vi "AutoCrossSubVi.vi"(0 "AutoDriveSpeed":dbl, 1 "DistanceAutoLineToBar":dbl, 2 "BarToShootLine":dbl, 3 "DriveDistanceDeadband":dbl, 5 "DriveDistanceVDeadband":dbl, 7 "VDeadband":dbl, 9 "EncoderDevRef 2":T1, 12 "Deadband":dbl, 13 "String":string, 14 "EncoderDevRef":T1) -> ()   [LabVIEW 2015]
uses:
  AutoTask/Implementation/AutoTask Operations.ctl
  AutoTask/Implementation/AutoTask Setpoints.ctl
  <vilib>/Rock Robotics/SystemInterfaces/Encoder/FPGA_EncoderIdx.ctl
  <vilib>/Rock Robotics/WPI/Encoder/WPI_EncoderType.ctl
  <vilib>/Rock Robotics/SystemInterfaces/Counter/FPGA_CounterCtrSystemIndex.ctl
  <vilib>/Rock Robotics/WPI/Encoder/WPI_EncoderDevRef.ctl
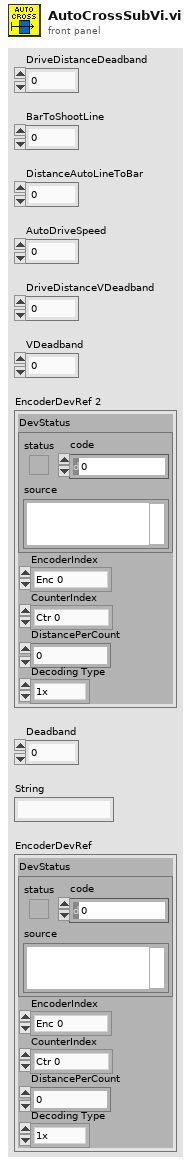
[diagram p1: front panel]
types:
  T1 = typedef "WPI_EncoderDevRef.ctl" = cluster{"DevStatus":errorcluster, "EncoderIndex":T2, "CounterIndex":T3, "DistancePerCount":dbl, "Decoding Type":T4}
  T2 = typedef "FPGA_EncoderIdx.ctl" = enum8{"Enc 0", "Enc 1", "Enc 2", "Enc 3", "Enc 4", "Enc 5", "Enc 6", "Enc 7", "Invalid"}
  T3 = typedef "FPGA_CounterCtrSystemIndex.ctl" = enum8{"Ctr 0", "Ctr 1", "Ctr 2", "Ctr 3", "Ctr 4", "Ctr 5", "Ctr 6", "Ctr 7", "Invalid"}
  T4 = typedef "WPI_EncoderType.ctl" = enum16{"1x", "2x", "4x"}
  T5 = typedef "AutoTask Setpoints.ctl" = cluster{"Operation":T6, "Setpoint":dbl, "Duration":dbl, "Speed":dbl, "Angle":dbl, "VDeadband":dbl, "Deadband":dbl, "DriveSpeed":dbl}
  T6 = typedef "AutoTask Operations.ctl" = enum16{"Reserve", "Read Current", "Immediate", "DriveDistance", "AutoShoot", "FaceForward", "AutoAlign", "AutoTurn", "DriveToLine", "DriveToIncline", "DriveTillFlat"}
  T7 = typedef "AutoTask Setpoints.ctl" = cluster{"Operation":T6, "Setpoint":dbl, "Duration":dbl, "Speed":dbl, "Angle":dbl, "VDeadband":dbl, "Deadband":dbl}
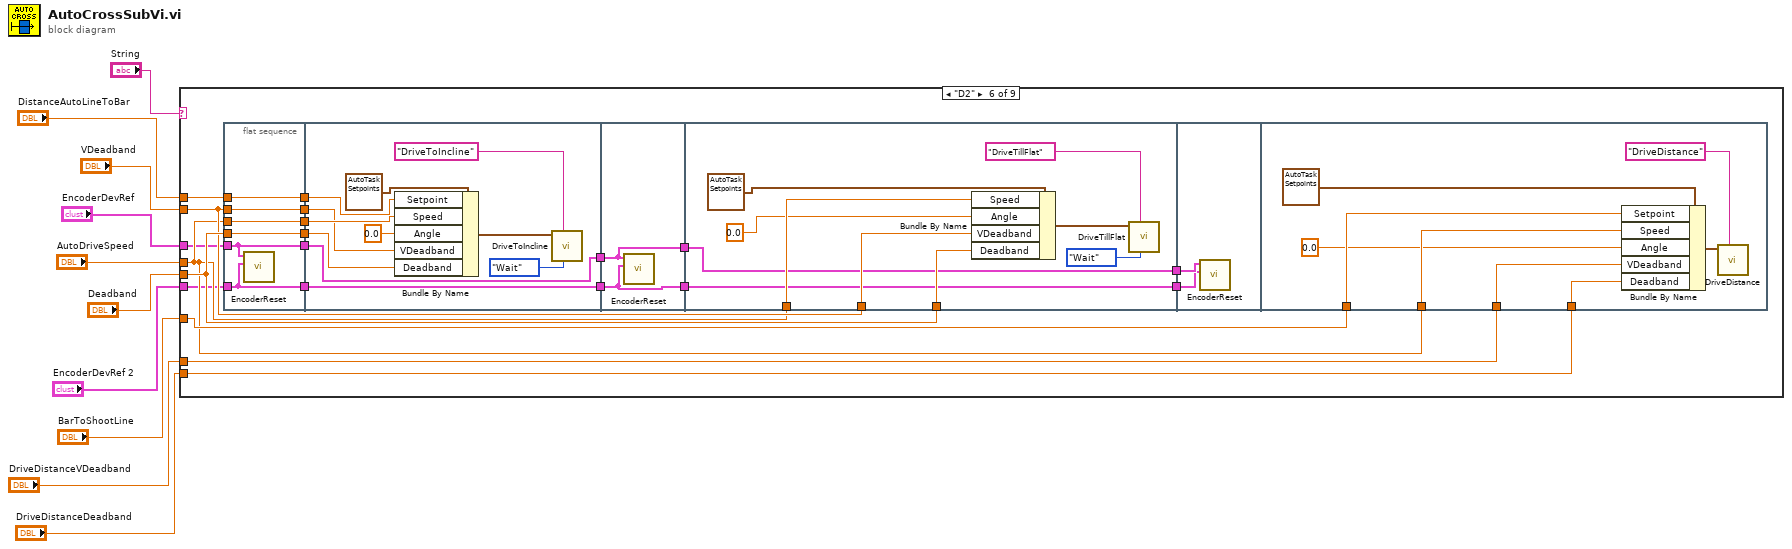
[diagram p0: block diagram]
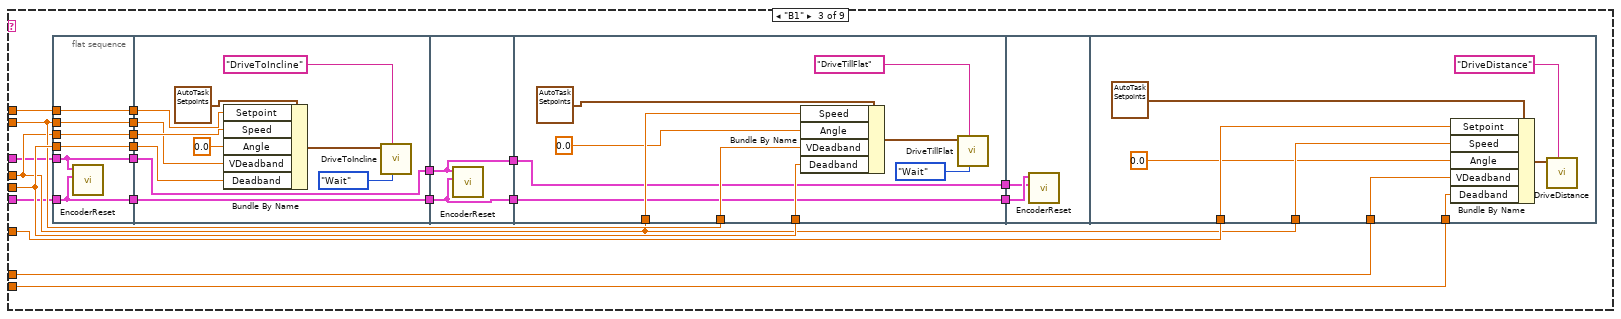
[diagram p4: hidden frame]
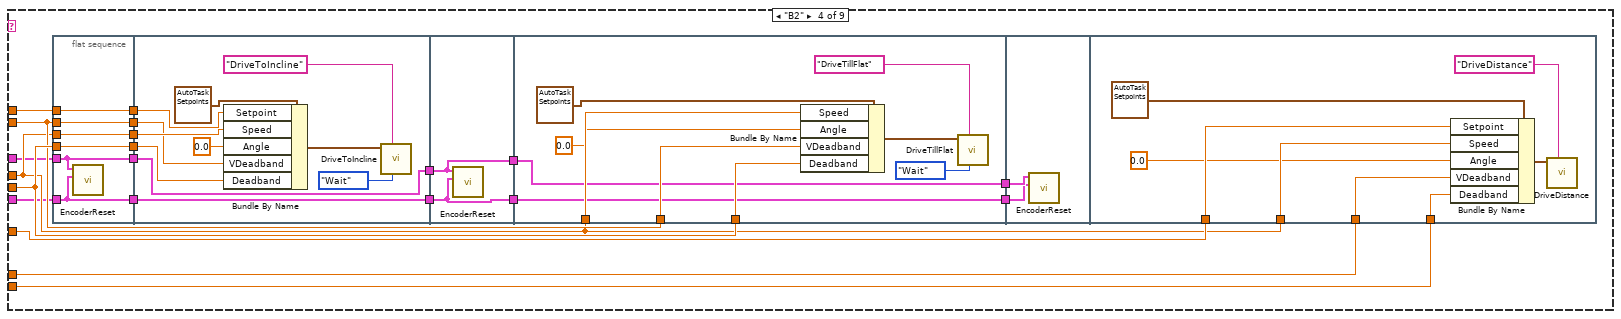
[diagram p5: hidden frame]
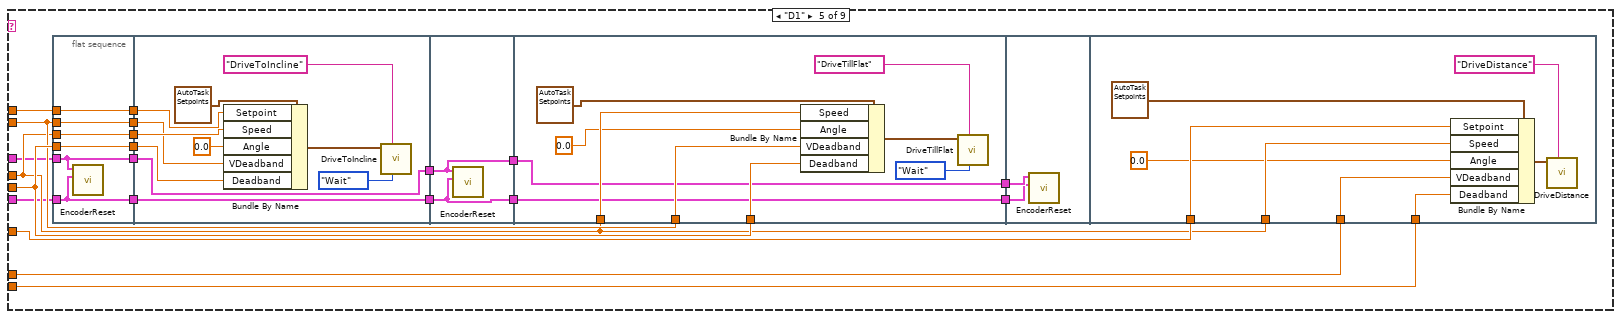
[diagram p6: hidden frame]
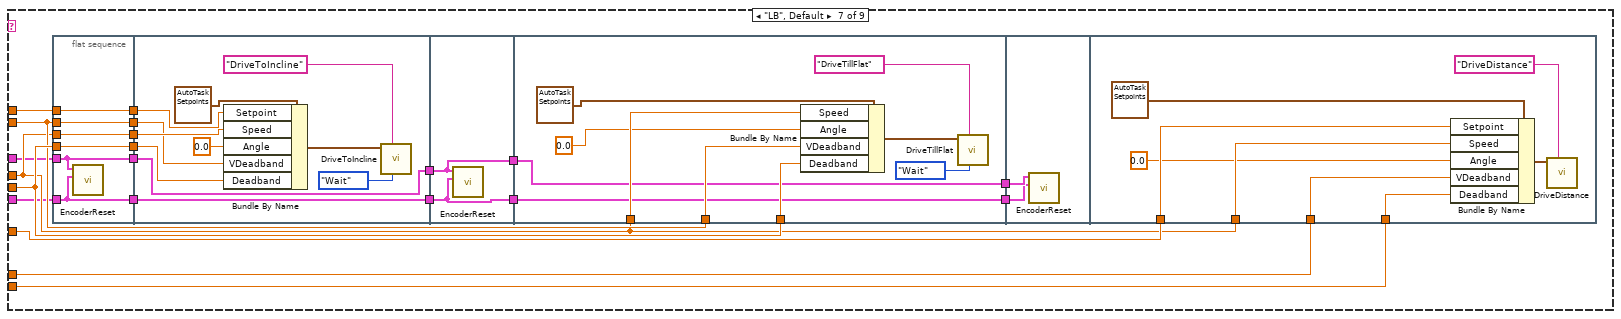
[diagram p7: hidden frame]
diagram:
  n1 = case shown="\"D2\"" "String" {
    tunnel: "DistanceAutoLineToBar" -> [_ _ w31 w91 w151 w211 w271 _ _]
    tunnel: "AutoDriveSpeed" -> [_ _ w27 w87 w147 w207 w267 _ _]
    tunnel: "VDeadband" -> [_ _ w29 w89 w149 w209 w269 _ _]
    tunnel: "Deadband" -> [_ _ w30 w90 w150 w210 w270 _ _]
    tunnel: "BarToShootLine" -> [_ _ w28 w88 w148 w208 w268 _ _]
    tunnel: "DriveDistanceDeadband" -> [_ _ w26 w86 w146 w206 w266 _ _]
    tunnel: "DriveDistanceVDeadband" -> [_ _ w25 w85 w145 w205 w265 _ _]
    tunnel: "EncoderDevRef 2" -> [_ _ w19 w79 w140 w199 w259 _ _]
    tunnel: "EncoderDevRef" -> [_ _ w20 w80 w139 w200 w260 _ _]
    frame "A1" {
    }
    frame "A2" {
    }
    frame "B1" {
      n2 = flat-sequence {
        tunnel: w30 -> [w34]
        tunnel: w29 -> [w35]
        tunnel: w27 -> [w36]
        tunnel: w31 -> [w37]
        tunnel: [w37] -> w24
        tunnel: [w36] -> w23
        tunnel: [w35] -> w22
        tunnel: [w34] -> w21
        tunnel: w20 -> [w33]
        tunnel: w19 -> [w32]
        tunnel: [w33] -> w18
        tunnel: [w32] -> w16
        tunnel: w24 -> [w45]
        tunnel: w23 -> [w44]
        tunnel: w22 -> [w42]
        tunnel: w21 -> [w41]
        tunnel: w18 -> [w39]
        tunnel: [w39] -> w17
        tunnel: w16 -> [w38]
        tunnel: [w38] -> w15
        tunnel: w17 -> [w49]
        tunnel: w15 -> [w50]
        tunnel: [w50] -> w14
        tunnel: [w49] -> w12
        tunnel: w27 -> [w56]
        tunnel: w30 -> [w54]
        tunnel: w29 -> [w53]
        tunnel: w14 -> [w52]
        tunnel: [w52] -> w13
        tunnel: w12 -> [w51]
        tunnel: [w51] -> w11
        tunnel: w13 -> [w62]
        tunnel: w11 -> [w61]
        tunnel: w28 -> [w67]
        tunnel: w27 -> [w66]
        tunnel: w26 -> [w64]
        tunnel: w25 -> [w63]
        frame #0 {
          n3 = call "EncoderReset.vi"("EncoderDevRef 2"=w32, "EncoderDevRef"=w33) -> ()  [unwired: 10 in]
        }
        frame #1 {
          n4 = Bundle By Name(cluster=T5 {"Operation"=enum."DriveToIncline", "Setpoint"=0.0, "Duration"=0.0, "Speed"=0.0, "Angle"=0.0, "VDeadband"=0.0, "Deadband"=0.0, "DriveSpeed"=0.0} ("SubSystem Data"), "Setpoint"=w45, "Speed"=w44, "Angle"=0.0, "VDeadband"=w42, "Deadband"=w41) -> (w47:T5)
          n5 = call "DriveToIncline.vi"("Synchronization"=enum16{"Start", "Wait"}."Wait", "Description"="DriveToIncline", "SubSystem Data"=w47) -> ()  [unwired: 8 in, 1 out]
        }
        frame #2 {
          n6 = call "EncoderReset.vi"("EncoderDevRef 2"=w50, "EncoderDevRef"=w49) -> ()  [unwired: 10 in]
        }
        frame #3 {
          n7 = Bundle By Name(cluster=T7 {"Operation"=enum."Reserve", "Setpoint"=0.0, "Duration"=0.0, "Speed"=0.0, "Angle"=0.0, "VDeadband"=0.0, "Deadband"=0.0} ("SubSystem Data"), "Speed"=w56, "Angle"=0.0, "VDeadband"=w53, "Deadband"=w54) -> (w59:T7)
          n8 = call "DriveTillFlat.vi"("Synchronization"=enum16{"Start", "Wait"}."Wait", "Description"="DriveTillFlat", "SubSystem Data"=w59) -> ()  [unwired: 8 in, 1 out]
        }
        frame #4 {
          n9 = call "EncoderReset.vi"("EncoderDevRef 2"=w61, "EncoderDevRef"=w62) -> ()  [unwired: 10 in]
        }
        frame #5 {
          n10 = Bundle By Name(cluster=T5 {"Operation"=enum."DriveDistance", "Setpoint"=0.0, "Duration"=0.0, "Speed"=0.0, "Angle"=0.0, "VDeadband"=0.0, "Deadband"=0.0, "DriveSpeed"=0.0} ("SubSystem Data"), "Setpoint"=w67, "Speed"=w66, "Angle"=0.0, "VDeadband"=w63, "Deadband"=w64) -> (w69:T5)
          n11 = call "DriveDistance.vi"("Description"="DriveDistance", "SubSystem Data"=w69) -> ()  [unwired: 9 in, 1 out]
        }
      }
    }
    frame "B2" {
      n12 = flat-sequence {
        tunnel: w90 -> [w94]
        tunnel: w89 -> [w95]
        tunnel: w87 -> [w96]
        tunnel: w91 -> [w97]
        tunnel: [w97] -> w84
        tunnel: [w96] -> w83
        tunnel: [w95] -> w82
        tunnel: [w94] -> w81
        tunnel: w80 -> [w93]
        tunnel: w79 -> [w92]
        tunnel: [w93] -> w78
        tunnel: [w92] -> w76
        tunnel: w84 -> [w105]
        tunnel: w83 -> [w104]
        tunnel: w82 -> [w102]
        tunnel: w81 -> [w101]
        tunnel: w78 -> [w99]
        tunnel: [w99] -> w77
        tunnel: w76 -> [w98]
        tunnel: [w98] -> w75
        tunnel: w77 -> [w110]
        tunnel: w75 -> [w109]
        tunnel: [w110] -> w74
        tunnel: [w109] -> w72
        tunnel: w87 -> [w116]
        tunnel: w90 -> [w114]
        tunnel: w89 -> [w113]
        tunnel: w74 -> [w112]
        tunnel: [w112] -> w73
        tunnel: w72 -> [w111]
        tunnel: [w111] -> w71
        tunnel: w73 -> [w122]
        tunnel: w71 -> [w121]
        tunnel: w88 -> [w127]
        tunnel: w87 -> [w126]
        tunnel: w86 -> [w124]
        tunnel: w85 -> [w123]
        frame #0 {
          n13 = call "EncoderReset.vi"("EncoderDevRef 2"=w92, "EncoderDevRef"=w93) -> ()  [unwired: 10 in]
        }
        frame #1 {
          n14 = Bundle By Name(cluster=T5 {"Operation"=enum."DriveToIncline", "Setpoint"=0.0, "Duration"=0.0, "Speed"=0.0, "Angle"=0.0, "VDeadband"=0.0, "Deadband"=0.0, "DriveSpeed"=0.0} ("SubSystem Data"), "Setpoint"=w105, "Speed"=w104, "Angle"=0.0, "VDeadband"=w102, "Deadband"=w101) -> (w107:T5)
          n15 = call "DriveToIncline.vi"("Synchronization"=enum16{"Start", "Wait"}."Wait", "Description"="DriveToIncline", "SubSystem Data"=w107) -> ()  [unwired: 8 in, 1 out]
        }
        frame #2 {
          n16 = call "EncoderReset.vi"("EncoderDevRef 2"=w109, "EncoderDevRef"=w110) -> ()  [unwired: 10 in]
        }
        frame #3 {
          n17 = Bundle By Name(cluster=T7 {"Operation"=enum."Reserve", "Setpoint"=0.0, "Duration"=0.0, "Speed"=0.0, "Angle"=0.0, "VDeadband"=0.0, "Deadband"=0.0} ("SubSystem Data"), "Speed"=w116, "Angle"=0.0, "VDeadband"=w113, "Deadband"=w114) -> (w119:T7)
          n18 = call "DriveTillFlat.vi"("Synchronization"=enum16{"Start", "Wait"}."Wait", "Description"="DriveTillFlat", "SubSystem Data"=w119) -> ()  [unwired: 8 in, 1 out]
        }
        frame #4 {
          n19 = call "EncoderReset.vi"("EncoderDevRef 2"=w121, "EncoderDevRef"=w122) -> ()  [unwired: 10 in]
        }
        frame #5 {
          n20 = Bundle By Name(cluster=T5 {"Operation"=enum."DriveDistance", "Setpoint"=0.0, "Duration"=0.0, "Speed"=0.0, "Angle"=0.0, "VDeadband"=0.0, "Deadband"=0.0, "DriveSpeed"=0.0} ("SubSystem Data"), "Setpoint"=w127, "Speed"=w126, "Angle"=0.0, "VDeadband"=w123, "Deadband"=w124) -> (w129:T5)
          n21 = call "DriveDistance.vi"("Description"="DriveDistance", "SubSystem Data"=w129) -> ()  [unwired: 9 in, 1 out]
        }
      }
    }
    frame "D1" {
      n22 = flat-sequence {
        tunnel: w150 -> [w154]
        tunnel: w149 -> [w155]
        tunnel: w147 -> [w156]
        tunnel: w151 -> [w157]
        tunnel: [w157] -> w144
        tunnel: [w156] -> w143
        tunnel: [w155] -> w142
        tunnel: [w154] -> w141
        tunnel: w140 -> [w152]
        tunnel: w139 -> [w153]
        tunnel: [w153] -> w138
        tunnel: [w152] -> w137
        tunnel: w144 -> [w165]
        tunnel: w143 -> [w164]
        tunnel: w142 -> [w162]
        tunnel: w141 -> [w161]
        tunnel: w138 -> [w159]
        tunnel: w137 -> [w158]
        tunnel: [w159] -> w136
        tunnel: [w158] -> w135
        tunnel: w136 -> [w170]
        tunnel: w135 -> [w169]
        tunnel: [w170] -> w134
        tunnel: [w169] -> w132
        tunnel: w147 -> [w176]
        tunnel: w150 -> [w174]
        tunnel: w149 -> [w173]
        tunnel: w134 -> [w172]
        tunnel: [w172] -> w133
        tunnel: w132 -> [w171]
        tunnel: [w171] -> w131
        tunnel: w133 -> [w182]
        tunnel: w131 -> [w181]
        tunnel: w148 -> [w187]
        tunnel: w147 -> [w186]
        tunnel: w146 -> [w184]
        tunnel: w145 -> [w183]
        frame #0 {
          n23 = call "EncoderReset.vi"("EncoderDevRef 2"=w152, "EncoderDevRef"=w153) -> ()  [unwired: 10 in]
        }
        frame #1 {
          n24 = Bundle By Name(cluster=T5 {"Operation"=enum."DriveToIncline", "Setpoint"=0.0, "Duration"=0.0, "Speed"=0.0, "Angle"=0.0, "VDeadband"=0.0, "Deadband"=0.0, "DriveSpeed"=0.0} ("SubSystem Data"), "Setpoint"=w165, "Speed"=w164, "Angle"=0.0, "VDeadband"=w162, "Deadband"=w161) -> (w167:T5)
          n25 = call "DriveToIncline.vi"("Synchronization"=enum16{"Start", "Wait"}."Wait", "Description"="DriveToIncline", "SubSystem Data"=w167) -> ()  [unwired: 8 in, 1 out]
        }
        frame #2 {
          n26 = call "EncoderReset.vi"("EncoderDevRef 2"=w169, "EncoderDevRef"=w170) -> ()  [unwired: 10 in]
        }
        frame #3 {
          n27 = Bundle By Name(cluster=T7 {"Operation"=enum."Reserve", "Setpoint"=0.0, "Duration"=0.0, "Speed"=0.0, "Angle"=0.0, "VDeadband"=0.0, "Deadband"=0.0} ("SubSystem Data"), "Speed"=w176, "Angle"=0.0, "VDeadband"=w173, "Deadband"=w174) -> (w179:T7)
          n28 = call "DriveTillFlat.vi"("Synchronization"=enum16{"Start", "Wait"}."Wait", "Description"="DriveTillFlat", "SubSystem Data"=w179) -> ()  [unwired: 8 in, 1 out]
        }
        frame #4 {
          n29 = call "EncoderReset.vi"("EncoderDevRef 2"=w181, "EncoderDevRef"=w182) -> ()  [unwired: 10 in]
        }
        frame #5 {
          n30 = Bundle By Name(cluster=T5 {"Operation"=enum."DriveDistance", "Setpoint"=0.0, "Duration"=0.0, "Speed"=0.0, "Angle"=0.0, "VDeadband"=0.0, "Deadband"=0.0, "DriveSpeed"=0.0} ("SubSystem Data"), "Setpoint"=w187, "Speed"=w186, "Angle"=0.0, "VDeadband"=w183, "Deadband"=w184) -> (w189:T5)
          n31 = call "DriveDistance.vi"("Description"="DriveDistance", "SubSystem Data"=w189) -> ()  [unwired: 9 in, 1 out]
        }
      }
    }
    frame "D2" {
      n32 = flat-sequence {
        tunnel: w210 -> [w214]
        tunnel: w209 -> [w215]
        tunnel: w207 -> [w216]
        tunnel: w211 -> [w217]
        tunnel: [w217] -> w204
        tunnel: [w216] -> w203
        tunnel: [w215] -> w202
        tunnel: [w214] -> w201
        tunnel: w200 -> [w213]
        tunnel: w199 -> [w212]
        tunnel: [w213] -> w198
        tunnel: [w212] -> w196
        tunnel: w204 -> [w225]
        tunnel: w203 -> [w224]
        tunnel: w202 -> [w222]
        tunnel: w201 -> [w221]
        tunnel: w198 -> [w219]
        tunnel: [w219] -> w197
        tunnel: w196 -> [w218]
        tunnel: [w218] -> w195
        tunnel: w197 -> [w230]
        tunnel: w195 -> [w229]
        tunnel: [w230] -> w194
        tunnel: [w229] -> w192
        tunnel: w207 -> [w236]
        tunnel: w210 -> [w234]
        tunnel: w209 -> [w233]
        tunnel: w194 -> [w232]
        tunnel: [w232] -> w193
        tunnel: w192 -> [w231]
        tunnel: [w231] -> w191
        tunnel: w193 -> [w242]
        tunnel: w191 -> [w241]
        tunnel: w208 -> [w247]
        tunnel: w207 -> [w246]
        tunnel: w206 -> [w244]
        tunnel: w205 -> [w243]
        frame #0 {
          n33 = call "EncoderReset.vi"("EncoderDevRef 2"=w212, "EncoderDevRef"=w213) -> ()  [unwired: 10 in]
        }
        frame #1 {
          n34 = Bundle By Name(cluster=T5 {"Operation"=enum."DriveToIncline", "Setpoint"=0.0, "Duration"=0.0, "Speed"=0.0, "Angle"=0.0, "VDeadband"=0.0, "Deadband"=0.0, "DriveSpeed"=0.0} ("SubSystem Data"), "Setpoint"=w225, "Speed"=w224, "Angle"=0.0, "VDeadband"=w222, "Deadband"=w221) -> (w227:T5)
          n35 = call "DriveToIncline.vi"("Synchronization"=enum16{"Start", "Wait"}."Wait", "Description"="DriveToIncline", "SubSystem Data"=w227) -> ()  [unwired: 8 in, 1 out]
        }
        frame #2 {
          n36 = call "EncoderReset.vi"("EncoderDevRef 2"=w229, "EncoderDevRef"=w230) -> ()  [unwired: 10 in]
        }
        frame #3 {
          n37 = Bundle By Name(cluster=T7 {"Operation"=enum."Reserve", "Setpoint"=0.0, "Duration"=0.0, "Speed"=0.0, "Angle"=0.0, "VDeadband"=0.0, "Deadband"=0.0} ("SubSystem Data"), "Speed"=w236, "Angle"=0.0, "VDeadband"=w233, "Deadband"=w234) -> (w239:T7)
          n38 = call "DriveTillFlat.vi"("Synchronization"=enum16{"Start", "Wait"}."Wait", "Description"="DriveTillFlat", "SubSystem Data"=w239) -> ()  [unwired: 8 in, 1 out]
        }
        frame #4 {
          n39 = call "EncoderReset.vi"("EncoderDevRef 2"=w241, "EncoderDevRef"=w242) -> ()  [unwired: 10 in]
        }
        frame #5 {
          n40 = Bundle By Name(cluster=T5 {"Operation"=enum."DriveDistance", "Setpoint"=0.0, "Duration"=0.0, "Speed"=0.0, "Angle"=0.0, "VDeadband"=0.0, "Deadband"=0.0, "DriveSpeed"=0.0} ("SubSystem Data"), "Setpoint"=w247, "Speed"=w246, "Angle"=0.0, "VDeadband"=w243, "Deadband"=w244) -> (w249:T5)
          n41 = call "DriveDistance.vi"("Description"="DriveDistance", "SubSystem Data"=w249) -> ()  [unwired: 9 in, 1 out]
        }
      }
    }
    frame "LB", Default {
      n42 = flat-sequence {
        tunnel: w270 -> [w274]
        tunnel: w269 -> [w275]
        tunnel: w267 -> [w276]
        tunnel: w271 -> [w277]
        tunnel: [w277] -> w264
        tunnel: [w276] -> w263
        tunnel: [w275] -> w262
        tunnel: [w274] -> w261
        tunnel: w260 -> [w273]
        tunnel: w259 -> [w272]
        tunnel: [w273] -> w258
        tunnel: [w272] -> w256
        tunnel: w264 -> [w285]
        tunnel: w263 -> [w284]
        tunnel: w262 -> [w282]
        tunnel: w261 -> [w281]
        tunnel: w258 -> [w279]
        tunnel: [w279] -> w257
        tunnel: w256 -> [w278]
        tunnel: [w278] -> w255
        tunnel: w257 -> [w290]
        tunnel: w255 -> [w289]
        tunnel: [w290] -> w254
        tunnel: [w289] -> w252
        tunnel: w267 -> [w296]
        tunnel: w270 -> [w294]
        tunnel: w269 -> [w293]
        tunnel: w254 -> [w292]
        tunnel: [w292] -> w253
        tunnel: w252 -> [w291]
        tunnel: [w291] -> w251
        tunnel: w253 -> [w302]
        tunnel: w251 -> [w301]
        tunnel: w268 -> [w307]
        tunnel: w267 -> [w306]
        tunnel: w266 -> [w304]
        tunnel: w265 -> [w303]
        frame #0 {
          n43 = call "EncoderReset.vi"("EncoderDevRef 2"=w272, "EncoderDevRef"=w273) -> ()  [unwired: 10 in]
        }
        frame #1 {
          n44 = Bundle By Name(cluster=T5 {"Operation"=enum."DriveToIncline", "Setpoint"=0.0, "Duration"=0.0, "Speed"=0.0, "Angle"=0.0, "VDeadband"=0.0, "Deadband"=0.0, "DriveSpeed"=0.0} ("SubSystem Data"), "Setpoint"=w285, "Speed"=w284, "Angle"=0.0, "VDeadband"=w282, "Deadband"=w281) -> (w287:T5)
          n45 = call "DriveToIncline.vi"("Synchronization"=enum16{"Start", "Wait"}."Wait", "Description"="DriveToIncline", "SubSystem Data"=w287) -> ()  [unwired: 8 in, 1 out]
        }
        frame #2 {
          n46 = call "EncoderReset.vi"("EncoderDevRef 2"=w289, "EncoderDevRef"=w290) -> ()  [unwired: 10 in]
        }
        frame #3 {
          n47 = Bundle By Name(cluster=T7 {"Operation"=enum."Reserve", "Setpoint"=0.0, "Duration"=0.0, "Speed"=0.0, "Angle"=0.0, "VDeadband"=0.0, "Deadband"=0.0} ("SubSystem Data"), "Speed"=w296, "Angle"=0.0, "VDeadband"=w293, "Deadband"=w294) -> (w299:T7)
          n48 = call "DriveTillFlat.vi"("Synchronization"=enum16{"Start", "Wait"}."Wait", "Description"="DriveTillFlat", "SubSystem Data"=w299) -> ()  [unwired: 8 in, 1 out]
        }
        frame #4 {
          n49 = call "EncoderReset.vi"("EncoderDevRef 2"=w301, "EncoderDevRef"=w302) -> ()  [unwired: 10 in]
        }
        frame #5 {
          n50 = Bundle By Name(cluster=T5 {"Operation"=enum."DriveDistance", "Setpoint"=0.0, "Duration"=0.0, "Speed"=0.0, "Angle"=0.0, "VDeadband"=0.0, "Deadband"=0.0, "DriveSpeed"=0.0} ("SubSystem Data"), "Setpoint"=w307, "Speed"=w306, "Angle"=0.0, "VDeadband"=w303, "Deadband"=w304) -> (w309:T5)
          n51 = call "DriveDistance.vi"("Description"="DriveDistance", "SubSystem Data"=w309) -> ()  [unwired: 9 in, 1 out]
        }
      }
    }
    frame "C1" {
    }
    frame "C2" {
    }
  }
